vi "ArrayDevHeaderData.vi"(0 "Experiment.lvclass In":refnum<class "Experiment.lvclass">, 5 "ArrayFuncName":string, 9 "IndCourbe":i64, 11 "error in":errorcluster caption="entrée d'erreur (pas d'erreur)", 13 "chemin Data":path) -> (1 "ArrQdata":string[](array[string])=["RTêta;", "X&Y;"], 3 "ArrVarParsOut":string[][](array[string]), 4 "Experiment.lvclass Out":refnum<class "Experiment.lvclass">, 6 "ArrHeaderPar":string, 8 "DevId":i32, 10 "ArrNomDon":string[](array[string])=["RTêta;", "X&Y;"], 12 "Experiment Name":string, 14 "Array Size":i32, 15 "error out":errorcluster caption="sortie d'erreur")   [LabVIEW 2019, in "Experiment.lvclass"]
uses:
  Experiment.lvclass
  Experiment.lvclass/Experiment.ctl
  DevicesClass/BaseDevice/BaseDevice.lvclass/BaseDevice.ctl
  DevicesClass/BaseDevice/Accessor/SetBaseDataPath.vi
  DevicesClass/BaseDevice/BaseDevice.lvclass
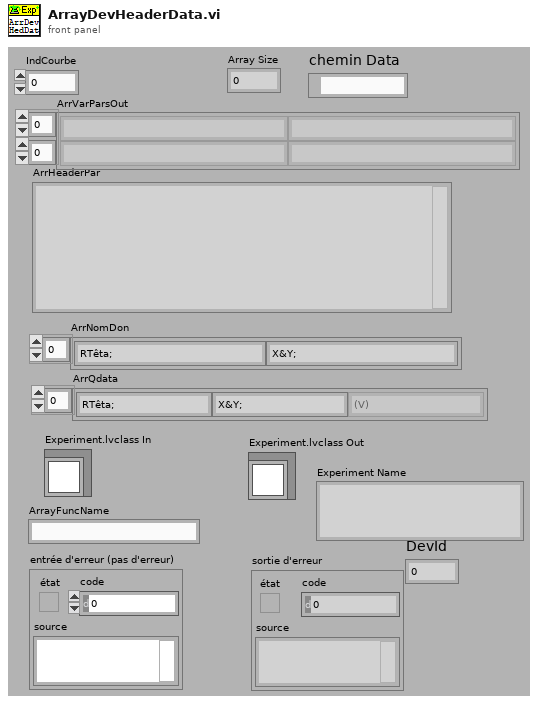
[diagram p1: front panel]
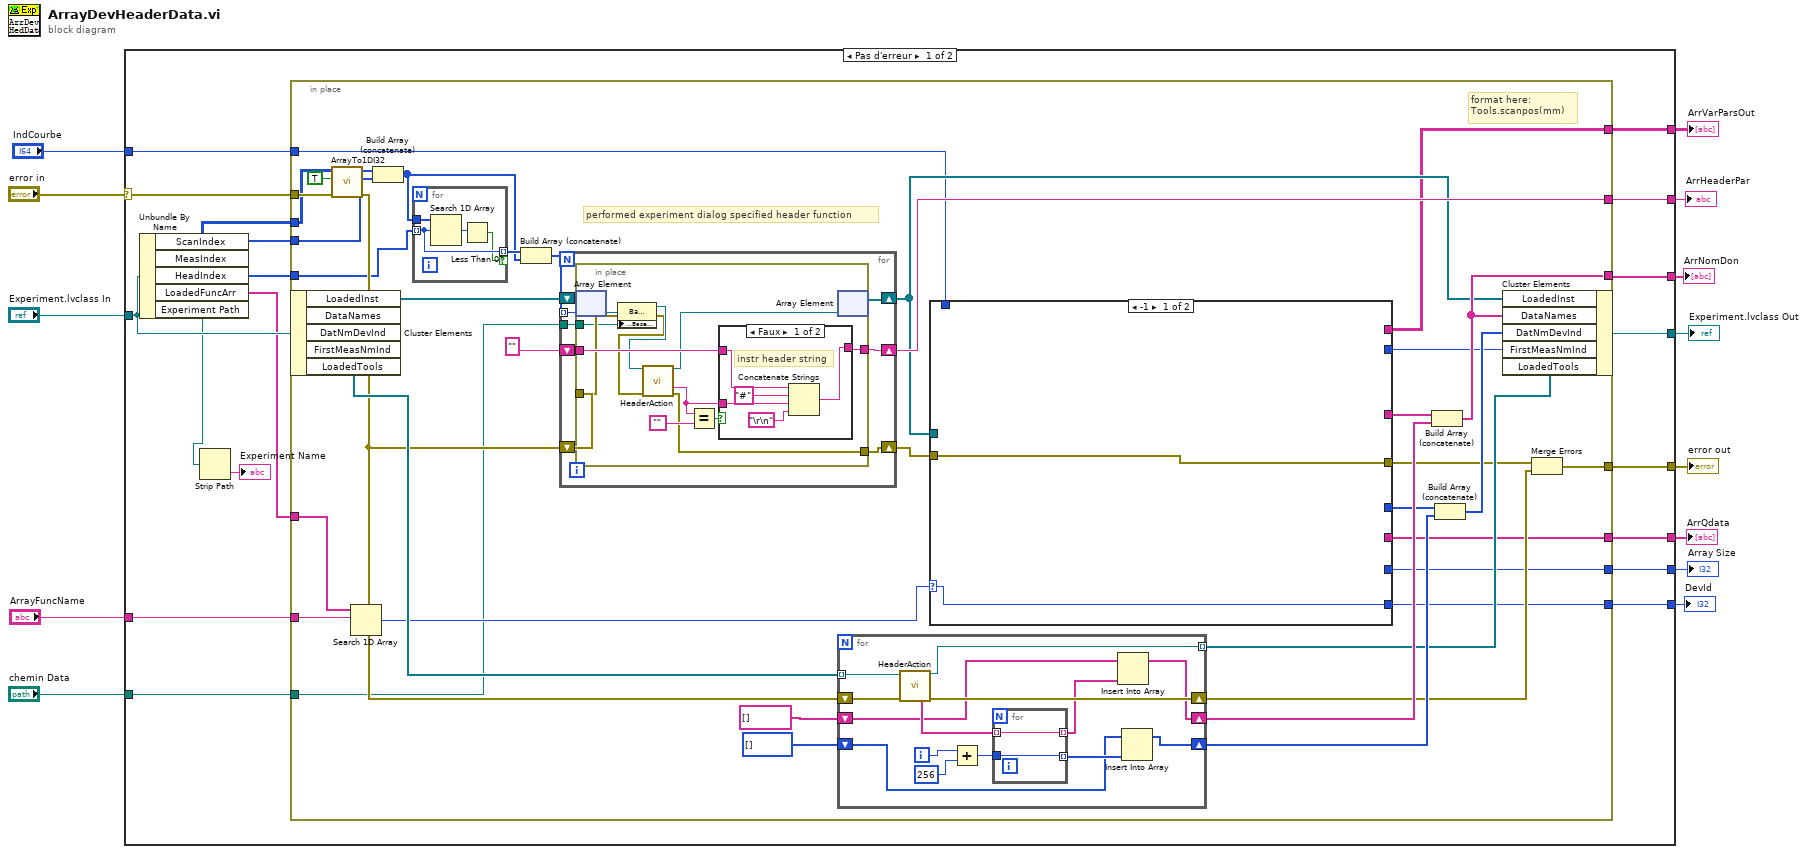
[diagram p0: block diagram]
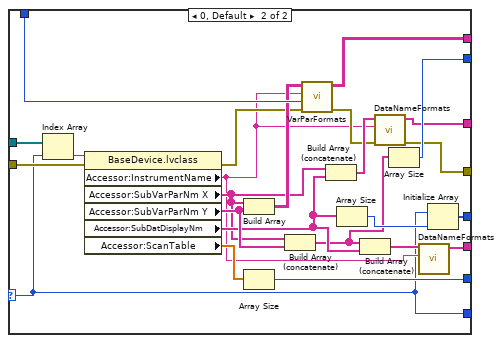
[diagram p2: hidden frame]
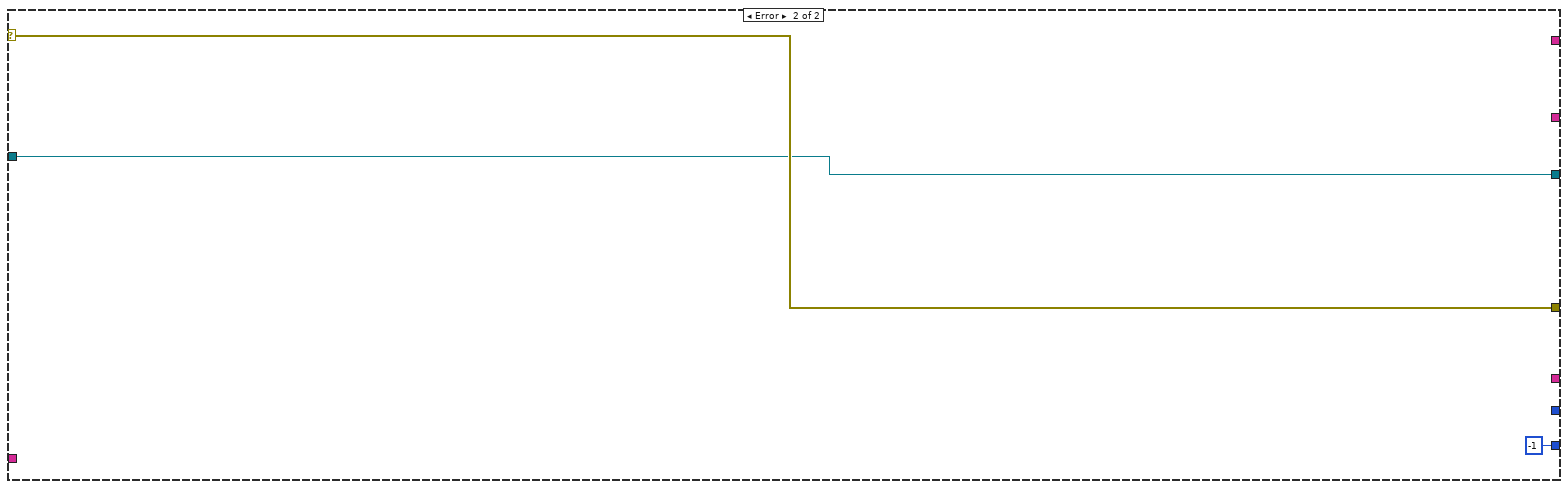
[diagram p4: hidden frame]
diagram:
  n1 = case shown="Pas d'erreur" "error in" {
    selector: "error in" -> [w27 w145]
    tunnel: [w23 w145] -> w12
    tunnel: [w32 _] -> w11
    tunnel: [w29 _] -> w10
    tunnel: "Experiment.lvclass In" -> [w31 w144]
    tunnel: [w30 w144] -> w8
    tunnel: "ArrayFuncName" -> [w24 _]
    tunnel: "IndCourbe" -> [w21 _]
    tunnel: [w20 _] -> w5
    tunnel: [w19 _] -> w4
    tunnel: [w18 _] -> w3
    tunnel: "chemin Data" -> [w15 _]
    tunnel: [w14 -1 ("index of element")] -> w1
    frame No Error {
      n2 = Unbundle By Name(w31) -> ("ScanIndex"=w28:i32[][], "MeasIndex"=w26:i32[], "HeadIndex"=w25:i32[], "LoadedFuncArr"=w22:string[], "Experiment Path"=w17:path)
      n3 = Strip Path(path=w17) -> (name=→"Experiment Name":string)  [unwired: 1 out]
      n4 = in-place {
        in-place-border: [w53] -> w32
        in-place-border: [w60] -> w29
        in-place-border: w27 -> [w68]
        in-place-border: [w46] -> w23
        in-place-border: w28 -> [w67]
        in-place-border: w26 -> [w57]
        in-place-border: w25 -> [w38]
        in-place-border: w22 -> [w55]
        in-place-border: w24 -> [w54]
        in-place-border: w21 -> [w43]
        in-place-border: [w40] -> w20
        in-place-border: [w41] -> w19
        in-place-border: [w39] -> w18
        in-place-border: w15 -> [w34]
        in-place-border: [w33] -> w14
        # "format here:\nTools.scanpos(mm)"
        # "performed experiment dialog specified header function"
        n5 = in-place-cluster #1(w31) -> ("LoadedInst"=w69:refnum<class "BaseDevice.lvclass">[], "LoadedTools"=w65:refnum<class "BaseDevice.lvclass">[])  [unwired: 3 out]
        n6 = call <userlib>:"ArrayTo1DI32.vi"("ErrorIn(No Error)"=w68, "DelArrEnd"=TRUE, "tableau"=w67) -> ("sortie d'erreur"=w44:errorcluster, "Array Out"=w56:i32[])  [unwired: 6 in, 1 out]
        n7 = Search 1D Array(1D array=w55, element=w54) -> (index of element=w50:i32)  [unwired: 1 in]
        n8 = Build Array (concatenate)(w56, w57) -> (w36:i32[])
        n9 = for {
          tunnel: w38 -> [w72] mode=indexing
          tunnel: w36 -> [w74]
          tunnel: [w72] -> w37 mode=indexing if=w71
          n10 = Search 1D Array(1D array=w74, element=w72) -> (index of element=w73:i32)  [unwired: 1 in]
          n11 = Less Than 0?(x=w73) -> (x < 0?=w71:bool)
        }
        n12 = Build Array (concatenate)(w37, w36) -> (w35:i32[])
        n13 = for {
          shift-right: [w106] -> w53
          shift-left: "" -> [w107]
          tunnel: w35 -> [w105] mode=indexing
          shift-right: [w103] -> w52
          shift-left: w69 -> [w104]
          shift-right: [w102] -> w51
          shift-left: w44 -> [w108]
          tunnel: w34 -> [w101]
          n14 = in-place {
            in-place-border: w108 -> [w111]
            in-place-border: w107 -> [w120]
            in-place-border: [w117] -> w102
            in-place-border: [w115] -> w106
            in-place-border: w101 -> [w109]
            n15 = in-place-array #2(w104, w105) -> (w114:refnum<class "BaseDevice.lvclass">)
            n16 = property class="BaseDevice.lvclass"(reference=w114, error in=w111, "Accessor:BaseDataPath"=w109) -> (reference out=w112:refnum<class "BaseDevice.lvclass">, error out=w110:errorcluster)
            n17 = call-dynamic "HeaderAction.vi"("Device en entrée"=w112, "error in (no error)"=w110) -> ("Device en sortie"=w113:refnum<class "BaseDevice.lvclass">, "HeaderString"=w116:string, "error out"=w117:errorcluster)  [unwired: 7 in, 4 out]
            n18 = Equal?(x=w116, y="") -> (x = y?=w119:bool)
            n19 = case shown="Faux" w119 {
              tunnel: [w124 w126] -> w115
              tunnel: w116 -> [w122 _]
              tunnel: w120 -> [w123 w126]
              frame False {
                # "instr header string"
                n20 = Concatenate Strings(w123, "#" ("chaîne"), w122, "\r\n") -> (w124:string)
              }
              frame True {
              }
            }
            n21 = in-place-array #2(w113) -> (w103:refnum<class "BaseDevice.lvclass">[])  [unwired: 1 out]
          }
        }
        n22 = for {
          tunnel: w65 -> [w140] mode=indexing
          shift-right: [w138] -> w45
          shift-left: w44 -> [w139]
          shift-right: [w130] -> w59
          shift-left: string[] [] -> [w132]
          shift-right: [w135] -> w61
          shift-left: i32[] [] -> [w134]
          tunnel: [w127] -> w58 mode=indexing
          i -> [w133]
          n23 = call-dynamic "HeaderAction.vi"("Device en entrée"=w140, "error in (no error)"=w139) -> ("Device en sortie"=w127:refnum<class "BaseDevice.lvclass">, "DisplayNames"=w137:string[], "error out"=w138:errorcluster)  [unwired: 7 in, 4 out]
          n24 = Add(x=w133, y=256) -> (x+y=w129:i32)
          n25 = for {
            tunnel: [w141] -> w131 mode=indexing
            tunnel: w129 -> [w142]
            tunnel: [w142] -> w136 mode=indexing
            tunnel: w137 -> [w141] mode=indexing
          }
          n26 = Insert Into Array(array=w132, new element=w131) -> (w130:string[])  [unwired: 1 in]
          n27 = Insert Into Array(array=w134, new element=w136) -> (w135:i32[])  [unwired: 1 in]
        }
        n28 = case shown="-1" w50 {
          selector: w50 -> [w75 w77]
          tunnel: w52 -> [_ w98]
          tunnel: w51 -> [w76 w99]
          tunnel: [w76 w81] -> w49
          tunnel: [_ w91] -> w48
          tunnel: [_ w83] -> w47
          tunnel: w43 -> [_ w96]
          tunnel: [_ w93] -> w40
          tunnel: [_ w89] -> w42
          tunnel: [_ w97] -> w41
          tunnel: [_ w79] -> w39
          tunnel: [w75 w77] -> w33
          frame -1 {
          }
          frame 0, Default {
            n29 = Index Array(array=w98, index=w77) -> (element=w100:refnum<class "BaseDevice.lvclass">)
            n30 = property class="BaseDevice.lvclass"(reference=w100, error in=w99) -> (error out=w94:errorcluster, "Accessor:InstrumentName"=w78:string, "Accessor:SubVarParNm X"=w86:string[], "Accessor:SubVarParNm Y"=w90:string[], "Accessor:SubDatDisplayNm"=w88:string[], "Accessor:ScanTable"=w92:dbl[])  [unwired: 1 out]
            n31 = Build Array(w86, w90) -> (w95:string[][])
            n32 = Array Size(array=w92) -> (size(s)=w97:i32)
            n33 = Build Array (concatenate)(w86, w90) -> (w85:string[])
            n34 = call "VarParFormats.vi"("ErrorIn(No Error)"=w94, "IndCourbe"=w96, "InstrumentName"=w78, "VarParArr"=w95) -> ("Err Out"=w82:errorcluster, "VarParArrOut"=w93:string[][])  [unwired: 6 in]
            n35 = Build Array (concatenate)(w86, w88) -> (w84:string[])
            n36 = Array Size(array=w88) -> (size(s)=w87:i32)
            n37 = Build Array (concatenate)(w85, w88) -> (w80:string[])
            n38 = call "DataNameFormats.vi"("ErrorIn(No Error)"=w82, "InstrumentName"=w78, "DataNameArr"=w84) -> ("Err Out"=w81:errorcluster, "DataNameArrOut"=w83:string[])  [unwired: 7 in]
            n39 = Array Size(array=w85) -> (size(s)=w89:i32)
            n40 = call "DataNameFormats.vi"("InstrumentName"=w78, "DataNameArr"=w80) -> ("DataNameArrOut"=w79:string[])  [unwired: 8 in, 1 out]
            n41 = Initialize Array(w77, w87) -> (w91:i32[])
          }
        }
        n42 = Build Array (concatenate)(w47, w59) -> (w60:string[])
        n43 = Build Array (concatenate)(w48, w61) -> (w62:i32[])
        n44 = in-place-cluster #1("LoadedInst"=w52, "DataNames"=w60, "DatNmDevInd"=w62, "FirstMeasNmInd"=w42, "LoadedTools"=w58) -> (w30:refnum<class "Experiment.lvclass">)
        n45 = Merge Errors(w49, w45) -> (w46:errorcluster)
      }
    }
    frame Error {
    }
  }
  "error out" <- w12
  "ArrHeaderPar" <- w11
  "ArrNomDon" <- w10
  "Experiment.lvclass Out" <- w8
  "ArrVarParsOut" <- w5
  "Array Size" <- w4
  "ArrQdata" <- w3
  "DevId" <- w1
